vi "Result.Parse Exec Rtn Data, STD OUT is code, Stderr is desc, Create Result Data_V1.vi"(7 "Name":string, 8 "BaseCode":i32, 9 "RtnCode":i32, 10 "StdErr":string, 11 "StdOut":string) -> (3 "Meas":T1[](array[typedef]) {"Status" items=["LOG", "PASS", "FAIL", "ERROR"]})   [LabVIEW 2018]
uses:
  Result.Measurement Item.ctl
  Result.Measurement and Attribute Item Status.ctl
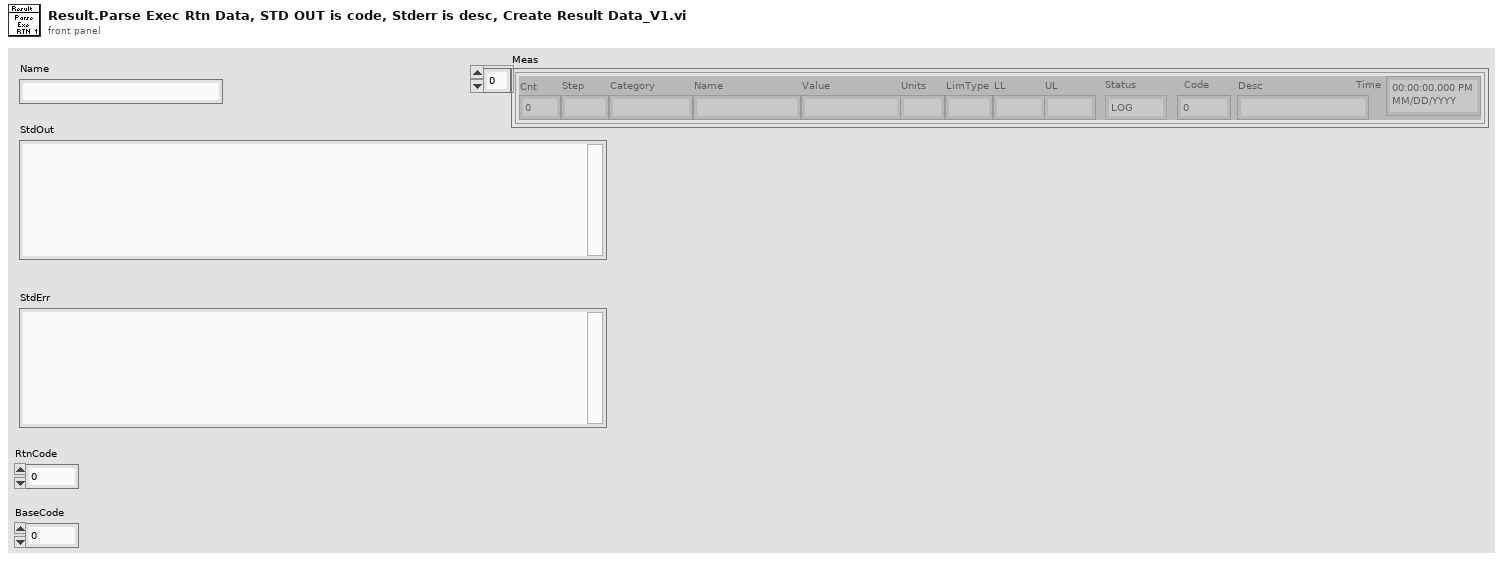
[diagram p1: front panel]
types:
  T1 = typedef "Result.Measurement Item.ctl" = cluster{"Cnt":i32, "Step":string, "Category":string, "Name":string, "Value":string, "Units":string, "LimType":string, "LL":string, "UL":string, "Status":T2, "Code":i32, "Desc":string, "Time":timestamp}
  T2 = typedef "Result.Measurement and Attribute Item Status.ctl" = i32
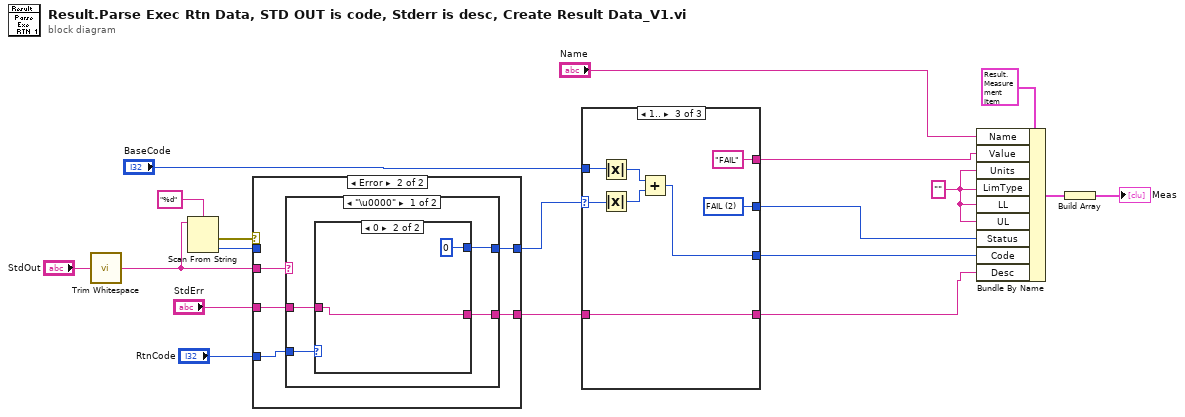
[diagram p0: block diagram]
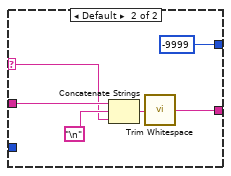
[diagram p4: hidden frame]
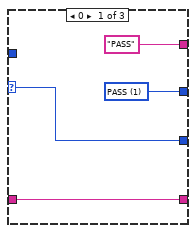
[diagram p5: hidden frame]
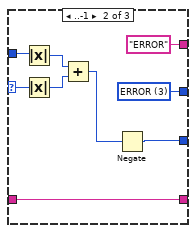
[diagram p6: hidden frame]
diagram:
  w14 = ""
  n1 = call <vilib>:"Trim Whitespace.vi"("string"="StdOut") -> ("trimmed string"=w5:string)  [unwired: 1 in]
  n2 = Scan From String(format string="%d", input string=w5) -> (error out=w8:errorcluster, output 1=w7:i32)  [unwired: 3 in, 2 out]
  n3 = case shown="Error" w8 {
    tunnel: w7 -> [w21 _]
    tunnel: [w21 w26] -> w6
    tunnel: w5 -> [_ w24]
    tunnel: "StdErr" -> [w20 w25]
    tunnel: [w20 w23] -> w3
    tunnel: "RtnCode" -> [_ w22]
    frame No Error {
    }
    frame Error {
      n4 = case shown="\"\"" w24 {
        selector: w24 -> [_ w37]
        tunnel: [w29 -9999] -> w26
        tunnel: w25 -> [w28 w38]
        tunnel: [w27 w35] -> w23
        tunnel: w22 -> [w30 _]
        frame "\u0000" {
          n5 = case shown="0" w30 {
            selector: w30 -> [w32 _]
            tunnel: [w32 0] -> w29
            tunnel: w28 -> [w31 w33]
            tunnel: [w31 w33] -> w27
            frame Default {
            }
            frame 0 {
            }
          }
        }
        frame Default {
          n6 = Concatenate Strings(w38, "\n", w37) -> (w36:string)
          n7 = call <vilib>:"Trim Whitespace.vi"("string"=w36) -> ("trimmed string"=w35:string)  [unwired: 1 in]
        }
      }
    }
  }
  n8 = case shown="1.." w6 {
    selector: w6 -> [w42 w51 w56]
    tunnel: [w44 w53 w61] -> w15
    tunnel: ["PASS" "ERROR" "FAIL"] -> w13
    tunnel: "BaseCode" -> [_ w50 w57]
    tunnel: [w42 w46 w55] -> w11
    tunnel: w3 -> [w41 w45 w54]
    tunnel: [w41 w45 w54] -> w2
    frame 0 {
      w44 = T2 1 items=["LOG", "PASS", "FAIL", "ERROR"] ("Status")
    }
    frame ..-1 {
      w53 = T2 3 items=["LOG", "PASS", "FAIL", "ERROR"] ("Status")
      n9 = Absolute Value(x=w50) -> (abs(x)=w49:i32)
      n10 = Absolute Value(x=w51) -> (abs(x)=w48:i32)
      n11 = Add(x=w49, y=w48) -> (x+y=w47:i32)
      n12 = Negate(x=w47) -> (-x=w46:i32)
    }
    frame 1.. {
      w61 = T2 2 items=["LOG", "PASS", "FAIL", "ERROR"] ("Status")
      n13 = Absolute Value(x=w57) -> (abs(x)=w59:i32)
      n14 = Absolute Value(x=w56) -> (abs(x)=w58:i32)
      n15 = Add(x=w59, y=w58) -> (x+y=w55:i32)
    }
  }
  n16 = Bundle By Name(cluster=T1 {"Cnt"=0, "Step"="", "Category"="", "Name"="", "Value"="", "Units"="", "LimType"="", "LL"="", "UL"="", "Status"=0, "Code"=0, "Desc"="", "Time"=timestamp(0 s since 1904-01-01)} ("Meas"), "Name"="Name", "Value"=w13, "Units"=w14, "LimType"=w14, "LL"=w14, "UL"=w14, "Status"=w15, "Code"=w11, "Desc"=w2) -> (w18:T1)
  n17 = Build Array(w18) -> (→"Meas":T1[])
